vi "Generate Waveform.vi"(0 "# Samples In":i32=128, 1 "Frequency/Sample Rate In":dbl, 2 "Index In":i32, 3 "Octave In":bool, 4 "Harmony In":bool) -> (5 "Audio Waveform Out":waveform(dbl), 6 "Graph Waveform Out":waveform(dbl))   [LabVIEW 2020]
doc: "Generate Waveform.vi takes in the Frequency/Sample Rate quotient that depends on the voltage read across the photoresistor and turns it into a waveform that can be played audially through speakers as well as a waveform that can be plotted on a waveform graph. It also adds a harmony and/or octave transposition to the waveform depending on whether either control is TRUE."
uses:
  <vilib>/Analysis/NI_AALBase.lvlib
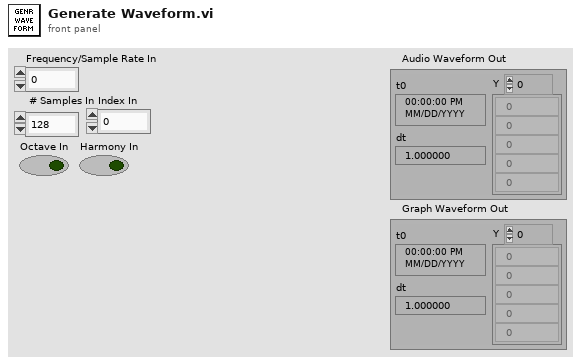
[diagram p1: front panel]
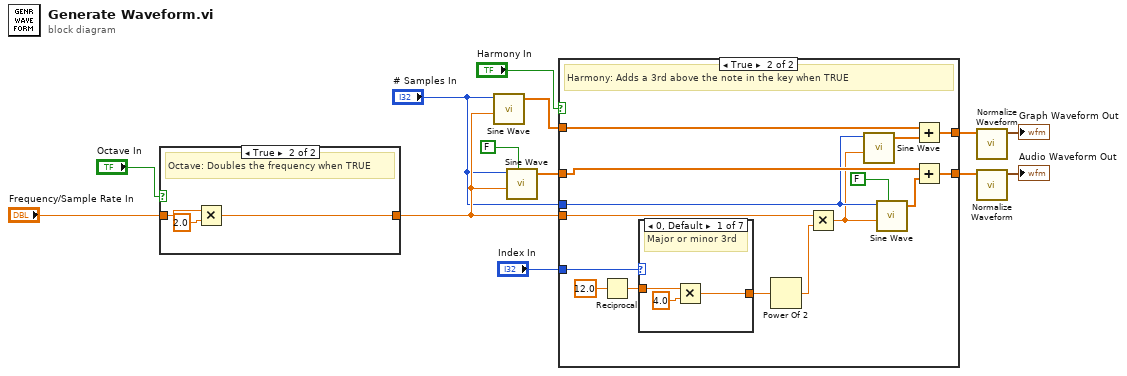
[diagram p0: block diagram]
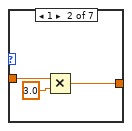
[diagram p4: hidden frame]
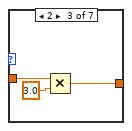
[diagram p5: hidden frame]
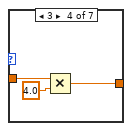
[diagram p6: hidden frame]
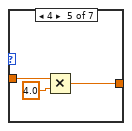
[diagram p7: hidden frame]
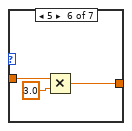
[diagram p8: hidden frame]
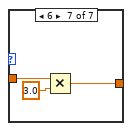
[diagram p9: hidden frame]
diagram:
  n1 = case shown="True" "Octave In" {
    tunnel: "Frequency/Sample Rate In" -> [w14 w16]
    tunnel: [w14 w15] -> w9
    frame False {
    }
    frame True {
      # "Octave: Doubles the frequency when TRUE"
      n2 = Multiply(x=w16, y=2.0) -> (x*y=w15:dbl)
    }
  }
  n3 = call <vilib>:"Sine Wave.vi"("samples"="# Samples In", "frequency"=w9) -> ("sine wave"=w8:dbl[])  [unwired: 3 in, 2 out]
  n4 = call <vilib>:"Sine Wave.vi"("samples"="# Samples In", "frequency"=w9, "reset phase"=FALSE) -> ("sine wave"=w12:dbl[])  [unwired: 2 in, 2 out]
  n5 = case shown="True" "Harmony In" {
    tunnel: "# Samples In" -> [_ w29]
    tunnel: w9 -> [_ w34]
    tunnel: w12 -> [w19 w32]
    tunnel: [w19 w31] -> w11
    tunnel: w8 -> [w18 w26]
    tunnel: [w18 w25] -> w7
    tunnel: "Index In" -> [_ w24]
    frame False {
    }
    frame True {
      # "Harmony: Adds a 3rd above the note in the key when TRUE"
      n6 = Reciprocal(x=12.0) -> (1/x=w22:dbl)
      n7 = case shown="0, Default" w24 {
        tunnel: [w36 w39 w42 w45 w48 w51 w54] -> w21
        tunnel: w22 -> [w37 w40 w43 w46 w49 w52 w55]
        frame 0, Default {
          # "Major or minor 3rd"
          n8 = Multiply(x=w37, y=4.0) -> (x*y=w36:dbl)
        }
        frame 1 {
          n9 = Multiply(x=w40, y=3.0) -> (x*y=w39:dbl)
        }
        frame 2 {
          n10 = Multiply(x=w43, y=3.0) -> (x*y=w42:dbl)
        }
        frame 3 {
          n11 = Multiply(x=w46, y=4.0) -> (x*y=w45:dbl)
        }
        frame 4 {
          n12 = Multiply(x=w49, y=4.0) -> (x*y=w48:dbl)
        }
        frame 5 {
          n13 = Multiply(x=w52, y=3.0) -> (x*y=w51:dbl)
        }
        frame 6 {
          n14 = Multiply(x=w55, y=3.0) -> (x*y=w54:dbl)
        }
      }
      n15 = Power Of 2(x=w21) -> (2^x=w20:dbl)
      n16 = Multiply(x=w34, y=w20) -> (x*y=w28:dbl)
      n17 = call <vilib>:"Sine Wave.vi"("samples"=w29, "frequency"=w28) -> ("sine wave"=w27:dbl[])  [unwired: 3 in, 2 out]
      n18 = call <vilib>:"Sine Wave.vi"("samples"=w29, "frequency"=w28, "reset phase"=FALSE) -> ("sine wave"=w30:dbl[])  [unwired: 2 in, 2 out]
      n19 = Add(x=w26, y=w27) -> (x+y=w25:dbl[])
      n20 = Add(x=w32, y=w30) -> (x+y=w31:dbl[])
    }
  }
  n21 = call <vilib>:"Normalize Waveform.vi"("waveform in"=w7) -> ("normalized waveform"=→"Graph Waveform Out":waveform(dbl))  [unwired: 7 in, 3 out]
  n22 = call <vilib>:"Normalize Waveform.vi"("waveform in"=w11) -> ("normalized waveform"=→"Audio Waveform Out":waveform(dbl))  [unwired: 7 in, 3 out]
